vi "Create_Image_From_Pixmap_Greyscale.vi"(8 "error in (no error)":errorcluster, 10 "Pixmap Image data":T1) -> (0 "error out":errorcluster, 3 "New Greyscale Image":refnum<data-value>)   [LabVIEW 2020, in "g_ar_toolkit.lvlib"]
uses:
  g_ar_toolkit.lvlib
  <vilib>/picture/picture.llb/imagedata.ctl
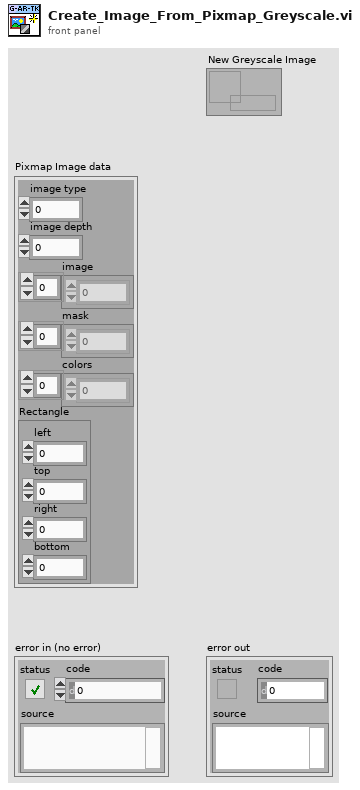
[diagram p1: front panel]
types:
  T1 = typedef "imagedata.ctl" = cluster{"image type":i32, "image depth":i32, "image":u8[], "mask":u8[], "colors":u32[], "Rectangle":cluster{"left":i16, "top":i16, "right":i16, "bottom":i16}}
  T2 = typedef "g_ar_toolkit.lvlib/Image Size Cluster.ctl" = cluster{"Width":u16, "Height":u16}
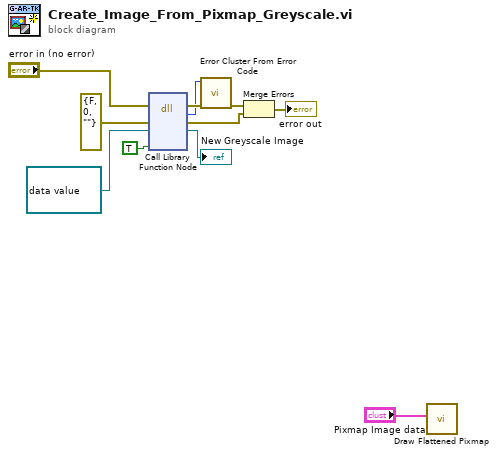
[diagram p0: block diagram]
diagram:
  n1 = dll-call lib="C:/serenial/libraries/g-augmented-reality-toolkit/LabVIEW/g_ar_toolkit/g_ar_toolkit.*.*" fn="Call Library Function Node"(error in="error in (no error)", "error_cluster"=errorcluster {"status"=FALSE, "code"=0, "source"=""} ("error constant"), "EDVR"=refnum<data-value> refnum, "is_bgra"=TRUE) -> (error out=w8:errorcluster, "MgErr"=w7:i32, "error_cluster"=w2:errorcluster, "EDVR"=→"New Greyscale Image":refnum<data-value>, "ImageSize"=w11:T2)  [unwired: 4 in, 1 out]
  n2 = call <vilib>:"Error Cluster From Error Code.vi"("error in (no error)"=w8, "error code (0)"=w7) -> ("error out"=w5:errorcluster)  [unwired: 7 in]
  n3 = Merge Errors(w5, w2) -> (→"error out":errorcluster)
  n4 = call <vilib>:"Draw Flattened Pixmap.vi"("image data"="Pixmap Image data") -> ()  [unwired: 8 in, 1 out]
